vi "Dereference.vi"(8 "error in (no error)":errorcluster, 11 "InstrPtr in":refnum<class "InstrPtr.lvclass">) -> (0 "error out":errorcluster, 2 "Instrument":refnum<class "Instrument.lvclass">, 3 "InstrPtr out":refnum<class "InstrPtr.lvclass">)   [LabVIEW 2009, in "InstrPtr.lvclass"]
doc: "The Instrument Pointer Class allows access to Instrument objects on the heap instead of on the stack. It accesses them in a thread-safe manner by using an internal reference queue. In other words, multiple programs can share the same Instrument class and read/write to the same variables, which keeps all references to the Instrument in sync with one another.\n\nSee LabVIEW\\examples\\lvoop\\ReferenceObject for details.\n\nDereference: this \"checks out\" the object, which you can then mutate with the standard accessor methods for the class. All other programs will wait (block) on this method until you check the object back in.\n\nReference: this \"checks in\" the object when you are done with it. Other classes will wait (block) to use the instrument until you check it back in."
uses:
  InstrPtr.lvclass
  Instrument/Instrument.lvclass
  InstrPtr.lvclass/InstrPtr.ctl
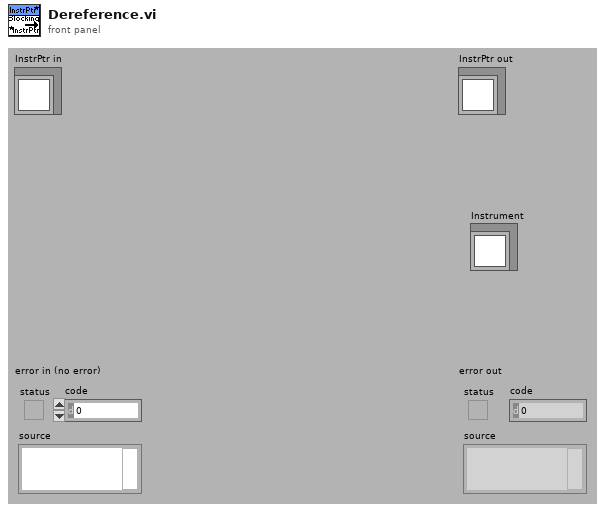
[diagram p1: front panel]
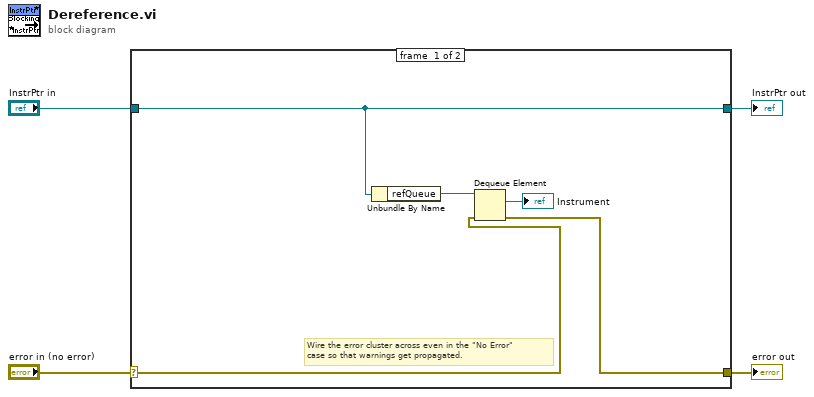
[diagram p0: block diagram]
diagram:
  n1 = case shown="No Error" "error in (no error)" {
    selector: "error in (no error)" -> [w6 w11]
    tunnel: [w5 w11] -> w3
    tunnel: [w8 w10] -> w1
    tunnel: "InstrPtr in" -> [w8 w10]
    frame #0 {
      # "Wire the error cluster across even in the \"No Error\"\ncase so that warnings get propagated."
      n2 = Unbundle By Name(w8) -> ("refQueue"=w9:refnum<queue>)
      n3 = Dequeue Element(queue=w9, error in (no error)=w6) -> (element=→"Instrument":refnum<class "Instrument.lvclass">, error out=w5:errorcluster)  [unwired: 3 out]
    }
    frame #1 {
    }
  }
  "error out" <- w3
  "InstrPtr out" <- w1
